vi "Configure Bus Controller Schedule.vi"(8 "error in (no error)":errorcluster) -> (0 "error out":errorcluster, 3 "Major Frame (Scheduled)":refnum<class "Major Frame.lvclass">)   [LabVIEW 2020, in "BCI-1553 RealTime API Examples.lvlib"]
uses:
  BCI-1553 RealTime API Examples.lvlib
  src/RealTime/Frames & Messages/Major Frame/Major Frame.lvclass
  src/RealTime/Frames & Messages/TypeDefs/Message Config.ctl
  src/RealTime/Frames & Messages/TypeDefs/Command Config.ctl
  src/RealTime/Frames & Messages/TypeDefs/Command Type.ctl
  src/RealTime/Frames & Messages/TypeDefs/Command Terminal Address.ctl
  src/RealTime/Frames & Messages/TypeDefs/Command SubAddress.ctl
  src/RealTime/Frames & Messages/TypeDefs/Command Word Count.ctl
  src/RealTime/Frames & Messages/TypeDefs/Message Control.ctl
  src/RealTime/Frames & Messages/TypeDefs/Simplified Parameter Data Table.ctl
  src/RealTime/Frames & Messages/TypeDefs/Scaling Information.ctl
  src/RealTime/Frames & Messages/Message/Message.lvclass
  src/RealTime/BCI-1553 API.lvlib
  src/RealTime/Frames & Messages/Minor Frame/Minor Frame.lvclass
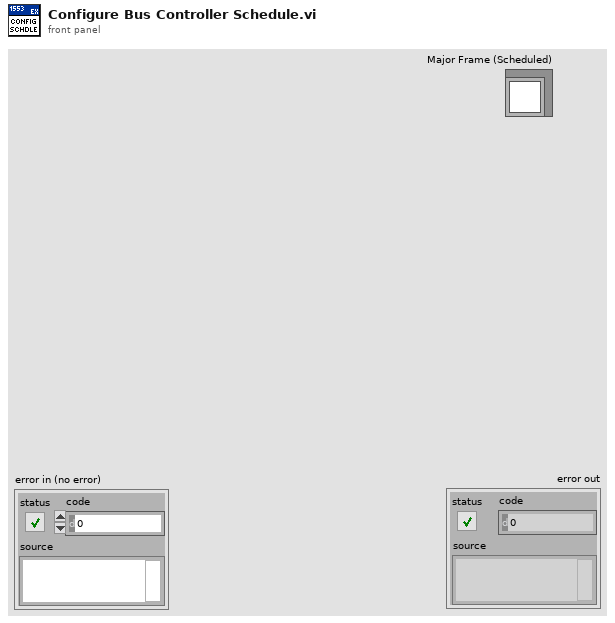
[diagram p1: front panel]
types:
  T1 = typedef "BCI-1553 API.lvlib/Simplified Parameter Data Table.ctl" = cluster{"Parameter Name":string, "Base Word":u16, "Scaling Info":T2}
  T2 = typedef "BCI-1553 API.lvlib/Scaling Information.ctl" = cluster{"Bit Offset":i32, "Bit Count":i32, "LSB Resolution":dbl, "2's Complement":bool, "Big Endian":bool, "Sign Bit":bool}
  T3 = typedef "BCI-1553 API.lvlib/Message Control.ctl" = cluster{"MC17 Time Sync":bool, "Error Mask":bool, "Service Request Mask":bool, "Busy Mask":bool, "SubSystem Flag Mask":bool, "Terminal Flag Mask":bool, "Reserved Mask":bool, "Retry":bool, "Bus A / !Bus B":bool, "Self-Test Loopback":bool, "Broadcast Mask":bool, "EoM Interrupt":bool, "Mode Code Format":bool, "Broadcast Format":bool, "RT-RT Format":bool}
  T4 = typedef "BCI-1553 API.lvlib/Command Word Count.ctl" = enum16{"1", "2", "3", "4", "5", "6", "7", "8", "9", "10", "11", "12", "13", "14", "15", "16", "17", "18", "19", "20", "21", "22", "23", "24", "25", "26", "27", "28", "29", "30", "31", "32"}
  T5 = typedef "BCI-1553 API.lvlib/Command SubAddress.ctl" = enum16{"Mode Code", "1", "2", "3", "4", "5", "6", "7", "8", "9", "10", "11", "12", "13", "14", "15", "16", "17", "18", "19", "20", "21", "22", "23", "24", "25", "26", "27", "28", "29", "30"}
  T6 = typedef "BCI-1553 API.lvlib/Command Terminal Address.ctl" = enum16{"0", "1", "2", "3", "4", "5", "6", "7", "8", "9", "10", "11", "12", "13", "14", "15", "16", "17", "18", "19", "20", "21", "22", "23", "24", "25", "26", "27", "28", "29", "30", "Broadcast"}
  T7 = typedef "BCI-1553 API.lvlib/Command Type.ctl" = enum16{"Transmit", "Receive"}
  T8 = typedef "BCI-1553 API.lvlib/Message Config.ctl" = cluster{"Time to Next Msg (4 us)":u16, "Command Config":T9, "Message Control":T3}
  T9 = typedef "BCI-1553 API.lvlib/Command Config.ctl" = cluster{"Command Type":T7, "Terminal Address":T6, "SubAddress":T5, "Word Count\\Mode Code":T4, "Command Data":u16[]}
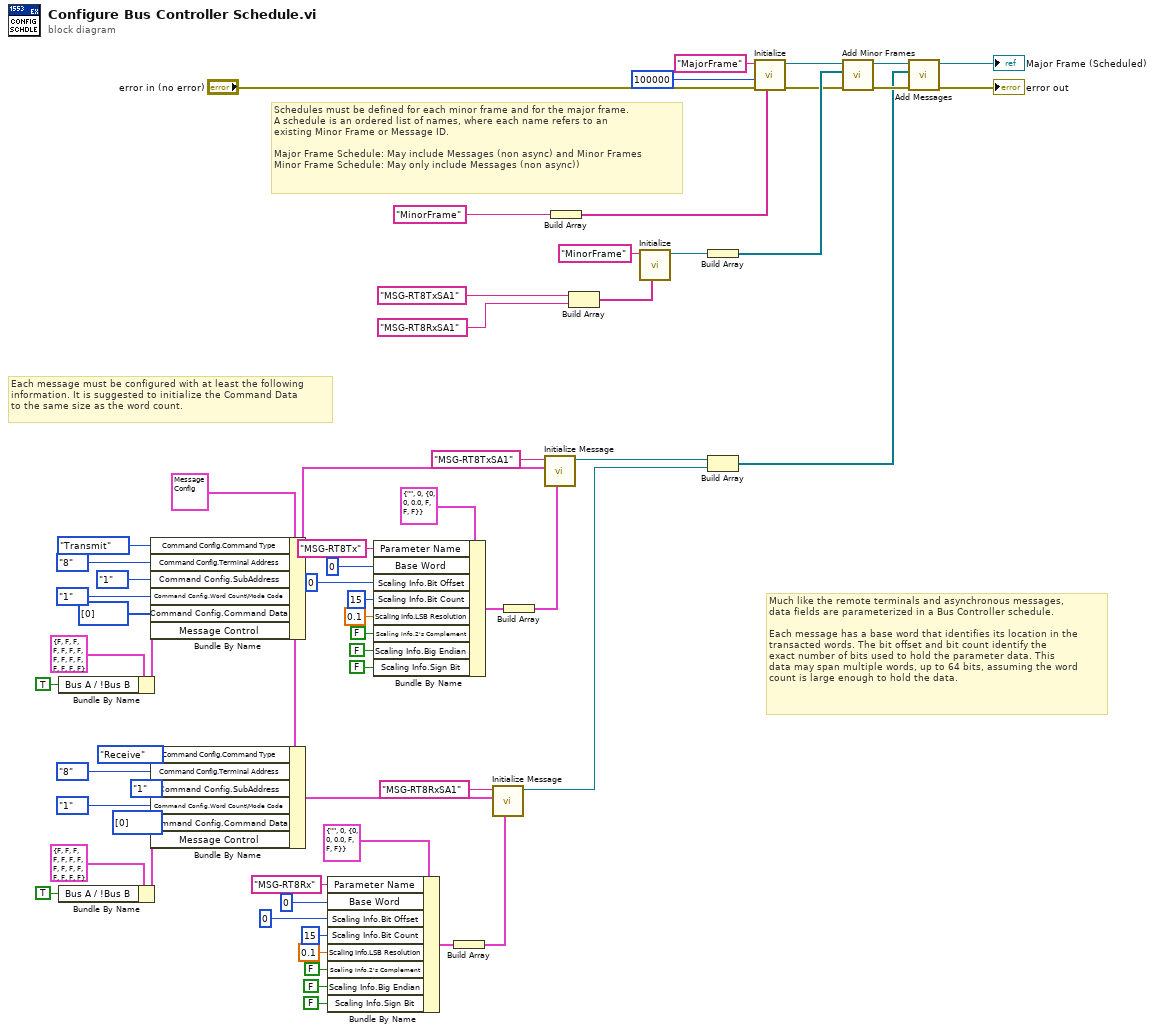
[diagram p0: block diagram]
diagram:
  w43 = T8 {"Time to Next Msg (4 us)"=100, "Command Config"={"Command Type"=enum."Transmit", "Terminal Address"=enum."0", "SubAddress"=enum."1", "Word Count\\Mode Code"=enum."1", "Command Data"=[]}, "Message Control"={"MC17 Time Sync"=FALSE, "Error Mask"=FALSE, "Service Request Mask"=FALSE, "Busy Mask"=FALSE, "SubSystem Flag Mask"=FALSE, "Terminal Flag Mask"=FALSE, "Reserved Mask"=FALSE, "Retry"=FALSE, "Bus A / !Bus B"=FALSE, "Self-Test Loopback"=FALSE, "Broadcast Mask"=FALSE, "EoM Interrupt"=FALSE, "Mode Code Format"=FALSE, "Broadcast Format"=FALSE, "RT-RT Format"=FALSE}} ("Message  Config")
  # "Each message must be configured with at least the following\ninformation. It is suggested to initialize the Command Data\nto the same size as the word count."
  # "Much like the remote terminals and asynchronous messages,\ndata fields are parameterized in a Bus Controller schedule.\n\nEach message has a base word that identifies its location in the\ntransacted words. The bit offset and bit count identify the\nexact number of bits used to hold the parameter data. This\ndata may span multiple words, up to 64 bits, assuming the word\ncount is large enough to hold the data."
  # "Schedules must be defined for each minor frame and for the major frame.\nA schedule is an ordered list of names, where each name refers to an\nexisting Minor Frame or Message ID.\n\nMajor Frame Schedule: May include Messages (non async) and Minor Frames\nMinor Frame Schedule: May only include Messages (non async))"
  n1 = Bundle By Name(cluster=T3 {"MC17 Time Sync"=FALSE, "Error Mask"=FALSE, "Service Request Mask"=FALSE, "Busy Mask"=FALSE, "SubSystem Flag Mask"=FALSE, "Terminal Flag Mask"=FALSE, "Reserved Mask"=FALSE, "Retry"=FALSE, "Bus A / !Bus B"=FALSE, "Self-Test Loopback"=FALSE, "Broadcast Mask"=FALSE, "EoM Interrupt"=FALSE, "Mode Code Format"=FALSE, "Broadcast Format"=FALSE, "RT-RT Format"=FALSE} ("Message Control"), "Bus A / !Bus B"=TRUE) -> (w54:T3)
  n2 = Bundle By Name(cluster=T3 {"MC17 Time Sync"=FALSE, "Error Mask"=FALSE, "Service Request Mask"=FALSE, "Busy Mask"=FALSE, "SubSystem Flag Mask"=FALSE, "Terminal Flag Mask"=FALSE, "Reserved Mask"=FALSE, "Retry"=FALSE, "Bus A / !Bus B"=FALSE, "Self-Test Loopback"=FALSE, "Broadcast Mask"=FALSE, "EoM Interrupt"=FALSE, "Mode Code Format"=FALSE, "Broadcast Format"=FALSE, "RT-RT Format"=FALSE} ("Message Control"), "Bus A / !Bus B"=TRUE) -> (w51:T3)
  n3 = Bundle By Name(cluster=w43, "Command Config.Command Type"=Command_Type."Transmit", "Command Config.Terminal Address"=Command_Terminal_Address."8", "Command Config.SubAddress"=Command_SubAddress."1", "Command Config.Word Count\\Mode Code"=Command_Word_Count."1" ("Command Config.Word Count"), "Command Config.Command Data"=u16[] [0], "Message Control"=w54) -> (w53:T8)
  n4 = Bundle By Name(cluster=w43, "Command Config.Command Type"=Command_Type."Receive", "Command Config.Terminal Address"=Command_Terminal_Address."8", "Command Config.SubAddress"=Command_SubAddress."1", "Command Config.Word Count\\Mode Code"=Command_Word_Count."1" ("Command Config.Word Count"), "Command Config.Command Data"=u16[] [0], "Message Control"=w51) -> (w42:T8)
  n5 = Bundle By Name(cluster=T1 {"Parameter Name"="", "Base Word"=0, "Scaling Info"={"Bit Offset"=0, "Bit Count"=0, "LSB Resolution"=0.0, "2's Complement"=FALSE, "Big Endian"=FALSE, "Sign Bit"=FALSE}} ("Parameters"), "Parameter Name"="MSG-RT8Rx", "Base Word"=u16 0, "Scaling Info.Bit Offset"=0, "Scaling Info.Bit Count"=15, "Scaling Info.LSB Resolution"=0.1, "Scaling Info.2's Complement"=FALSE, "Scaling Info.Big Endian"=FALSE, "Scaling Info.Sign Bit"=FALSE) -> (w29:T1)
  n6 = Bundle By Name(cluster=T1 {"Parameter Name"="", "Base Word"=0, "Scaling Info"={"Bit Offset"=0, "Bit Count"=0, "LSB Resolution"=0.0, "2's Complement"=FALSE, "Big Endian"=FALSE, "Sign Bit"=FALSE}} ("Parameters"), "Parameter Name"="MSG-RT8Tx", "Base Word"=u16 0, "Scaling Info.Bit Offset"=0, "Scaling Info.Bit Count"=15, "Scaling Info.LSB Resolution"=0.1, "Scaling Info.2's Complement"=FALSE, "Scaling Info.Big Endian"=FALSE, "Scaling Info.Sign Bit"=FALSE) -> (w41:T1)
  n7 = Build Array(w29) -> (w3:T1[])
  n8 = call "Initialize Message.vi"("Parameters"=w3, "Message  Config"=w42, "ID"="MSG-RT8RxSA1") -> ("Message out"=w16:refnum<class "Message.lvclass">)  [unwired: 7 in, 1 out]
  n9 = Build Array(w41) -> (w7:T1[])
  n10 = call "Initialize Message.vi"("Parameters"=w7, "Message  Config"=w53, "ID"="MSG-RT8TxSA1") -> ("Message out"=w17:refnum<class "Message.lvclass">)  [unwired: 7 in, 1 out]
  n11 = Build Array("MinorFrame" ("element")) -> (w12:string[])
  n12 = Build Array("MSG-RT8TxSA1" ("element"), "MSG-RT8RxSA1" ("element")) -> (w9:string[])
  n13 = call "Initialize.vi"("Schedule"=w9, "ID"="MinorFrame") -> ("Minor Frame out"=w24:refnum<class "Minor Frame.lvclass">)  [unwired: 8 in, 1 out]
  n14 = Build Array(w24) -> (w23:refnum<class "Minor Frame.lvclass">[])
  n15 = Build Array(w17, w16) -> (w15:refnum<class "Message.lvclass">[])
  n16 = call "Initialize.vi"("Schedule"=w12, "error in (no error)"="error in (no error)", "Minor Frame Time (100 us)"=u32 100000, "ID"="MajorFrame") -> ("error out"=w22:errorcluster, "Major Frame out"=w25:refnum<class "Major Frame.lvclass">)  [unwired: 6 in]
  n17 = call-dynamic "Add Minor Frames.vi"("error in (no error)"=w22, "Minor Frames"=w23, "Major Frame in"=w25) -> ("error out"=w19:errorcluster, "Major Frame out"=w20:refnum<class "Major Frame.lvclass">)  [unwired: 7 in]
  n18 = call-dynamic "Add Messages.vi"("error in (no error)"=w19, "Messages"=w15, "Major Frame in"=w20) -> ("error out"=→"error out":errorcluster, "Major Frame out"=→"Major Frame (Scheduled)":refnum<class "Major Frame.lvclass">)  [unwired: 7 in]
